vi "Main_11B_X3.vi"() -> ()   [LabVIEW 2024]
uses:
  Cluster_Blink result.ctl
  Utility/Universal Utility/TypeDefs_Utility/Cluster_Row-Column.ctl
panel:
  out "size(s)":i32
  in  "Example 2":string="125 17"
  in  "Use Puzzle":bool
  out "Answer 191690":u64
  in  "Puzzle":string="30 71441 3784 580926 2 8122942 0 291"
  in  "Example":string="0 1 10 99 999"
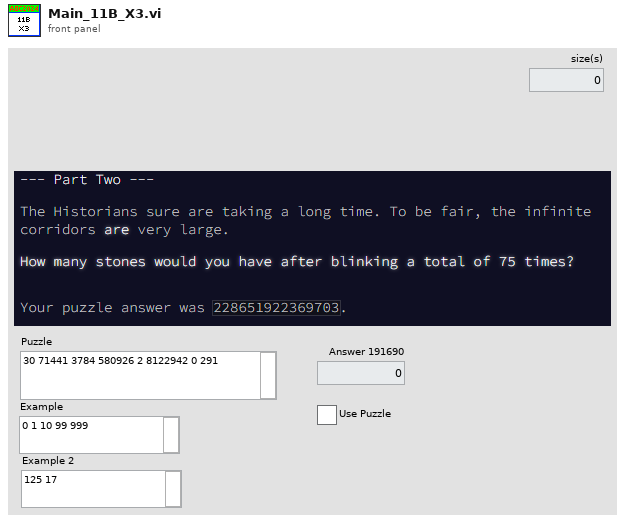
[diagram p1: front panel]
types:
  T1 = typedef "Cluster_Row-Column.ctl" = cluster{"R":i32, "C":i32}
  T2 = typedef "Cluster_Blink result.ctl" = cluster{"num":u64, "Blink":u64}
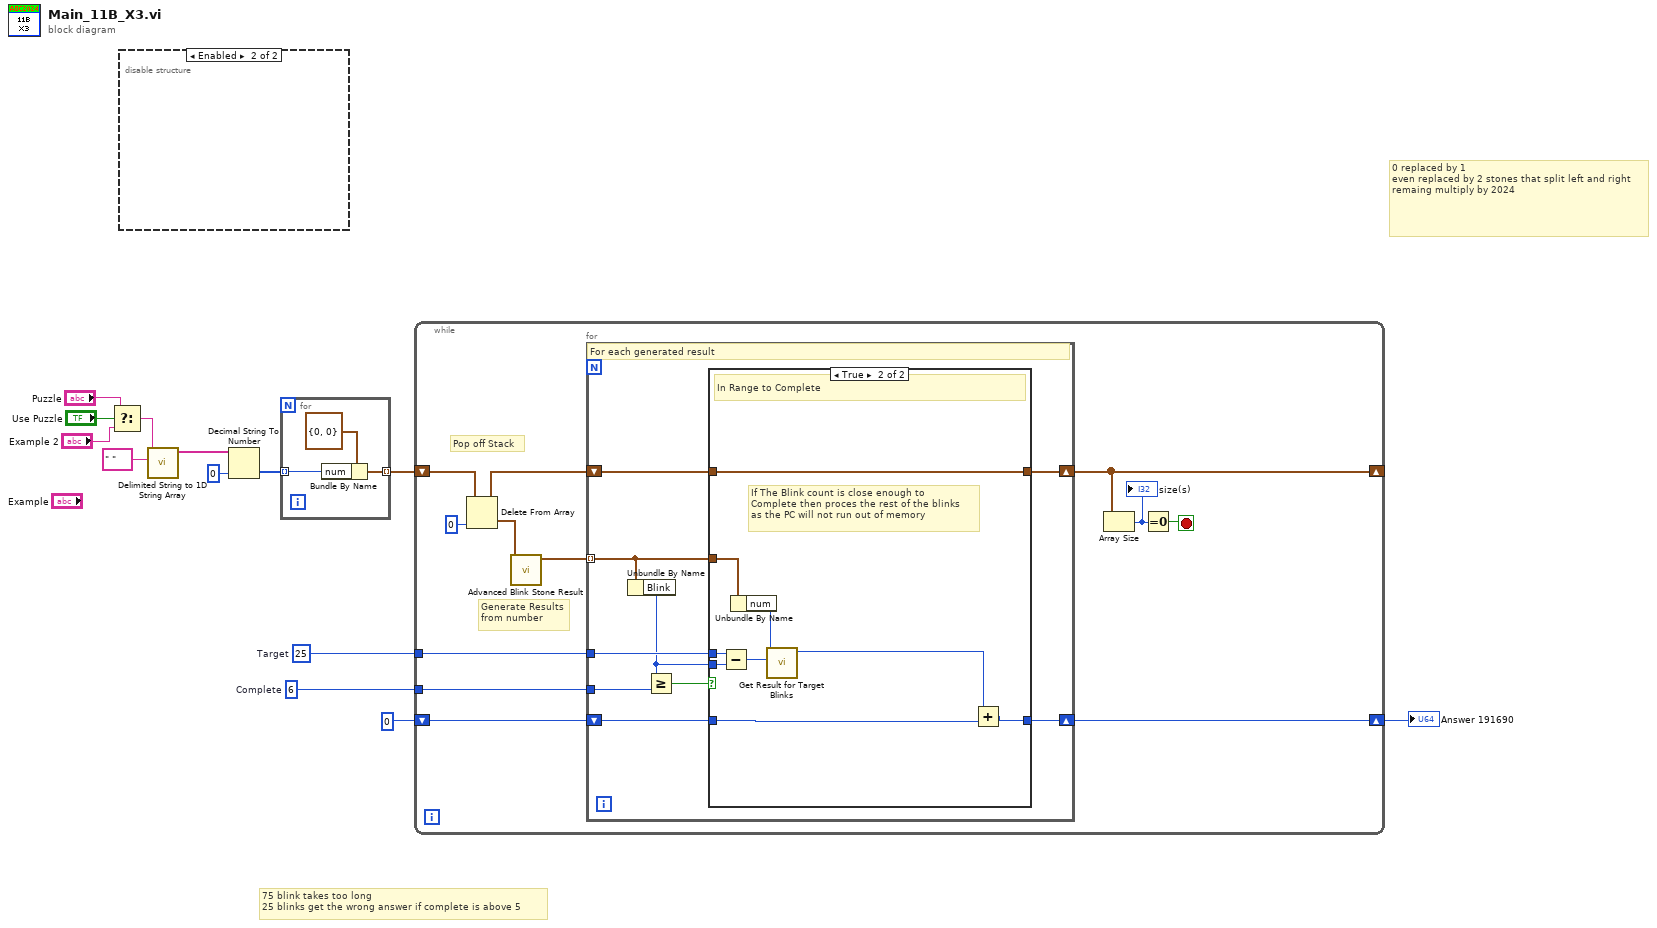
[diagram p0: block diagram]
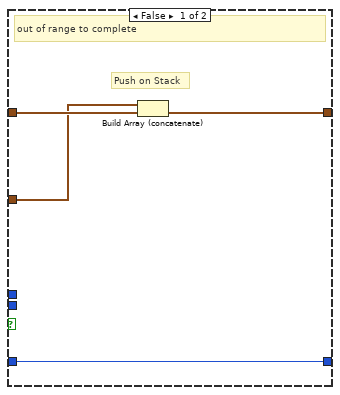
[diagram p2: hidden frame]
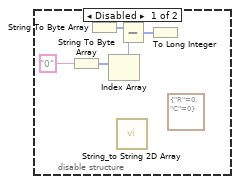
[diagram p3: hidden frame]
diagram:
  w1 = 6  # Complete
  w2 = 25  # Target
  # "75 blink takes too long\n25 blinks get the wrong answer if complete is above 5"
  # "0 replaced by 1\neven replaced by 2 stones that split left and right\nremaing multiply by 2024"
  n1 = Select(t="Puzzle", s="Use Puzzle", f="Example 2") -> (s? t:f=w11:string)
  n2 = disable-structure shown="Enabled" {
    frame Disabled {
      (unwired) T1 {"R"=0, "C"=0} ("Position")
      n3 = String To Byte Array(string="0") -> (unsigned byte array=w18:u8[])
      n4 = String To Byte Array() -> (string=w16:string, unsigned byte array=w15:u8[])
      n5 = Index Array(array=w18) -> (element=w17:u8)  [unwired: 1 in]
      n6 = call "String_to String 2D Array.vi"() -> ()  [unwired: 11 in, 1 out]
      n7 = Subtract(x=w15, y=w17) -> (x-y=w14:u8[])
      n8 = To Long Integer(number=w14) -> ()  [unwired: 1 out]
    }
    frame Enabled {
    }
  }
  n9 = call <vilib>:"Delimited String to 1D String Array.vi"("delimiter"=" " ("delimiter (Tab)"), "delimited string"=w11) -> ("string array"=w12:string[])  [unwired: 9 in]
  n10 = Decimal String To Number(string=w12, default (0L)=u64 0 ("default (0 I32)")) -> (number=w6:u64[])  [unwired: 1 in, 1 out]
  n11 = for {
    tunnel: w6 -> [w21] mode=indexing
    tunnel: [w20] -> w5 mode=indexing
    n12 = Bundle By Name(cluster=T2 {"num"=0, "Blink"=0} ("Result"), "num"=w21) -> (w20:T2)
  }
  n13 = while {
    shift-right: [w25] -> _
    shift-left: w5 -> [w34]
    tunnel: w2 -> [w26]
    shift-right: [w28] -> w3
    shift-left: u64 0 -> [w29]
    tunnel: w1 -> [w27]
    stop <- w23 stop-if-true
    # "Generate Results\nfrom number"
    # "Pop off Stack"
    n14 = Delete From Array(array=w34, index=0) -> (deleted portion=w32:T2, array with subset deleted=w30:T2[])  [unwired: 1 in]
    n15 = call "Advanced Blink Stone Result.vi"("Stone"=w32) -> ("Result Array"=w31:T2[])  [unwired: 10 in]
    n16 = for {
      tunnel: w31 -> [w42] mode=indexing
      shift-right: [w35] -> w25
      shift-left: w30 -> [w36]
      shift-right: [w37] -> w28
      shift-left: w29 -> [w38]
      tunnel: w27 -> [w43]
      tunnel: w26 -> [w40]
      # "For each generated result"
      n17 = Unbundle By Name(w42) -> ("Blink"=w39:u64)
      n18 = Greater Or Equal?(x=w39, y=w43) -> (x >= y?=w41:bool)
      n19 = case shown="True" w41 {
        tunnel: w42 -> [w46 w53]
        tunnel: w40 -> [_ w56]
        tunnel: w39 -> [_ w55]
        tunnel: w38 -> [w44 w51]
        tunnel: [w44 w50] -> w37
        tunnel: w36 -> [w47 w48]
        tunnel: [w45 w48] -> w35
        frame False {
          # "Push on Stack"
          # "out of range to complete"
          n20 = Build Array (concatenate)(w46, w47) -> (w45:T2[])
        }
        frame True {
          # "If The Blink count is close enough to \nComplete then proces the rest of the blinks\nas the PC will not run out of memory"
          # "In Range to Complete"
          n21 = Subtract(x=w56, y=w55) -> (x-y=w54:u64)
          n22 = Unbundle By Name(w53) -> ("num"=w52:u64)
          n23 = call "Get Result for Target Blinks.vi"("Target Blinks"=w54, "num"=w52) -> ("Count"=w49:i32)  [unwired: 9 in]
          n24 = Add(x=w49, y=w51) -> (x+y=w50:u64)
        }
      }
    }
    n25 = Array Size(array=w25) -> (size(s)=w24:i32)
    "size(s)" <- w24
    n26 = Equal To 0?(x=w24) -> (x = 0?=w23:bool)
  }
  "Answer 191690" <- w3
